vi "New motor Control integrated remodeled with PID.vi"(0 "States":enum16{"RESET ENCODER", "WRITE", "READ", "INIT"}(ring), 1 "Target Speed":T2 {"wTargetSpeed" scale=-1.0..1.0; "yTargetSpeed" scale=-1.0..1.0; "xTargetSpeed" scale=-1.0..1.0}, 3 "Error in":errorcluster) -> (5 "Speed and distance cluster":T1, 6 "Error out":errorcluster)   [LabVIEW 2018]
uses:
  <vilib>/addons/control/pid/pid.llb/PID (DBL).vi
  <vilib>/addons/control/pid/NI_PID_pid.lvlib
panel:
  out "output 3":dbl format="%.2f"
  out "output 2":dbl format="%.2f"
  out "output":dbl format="%.2f"
  out "output variable":dbl
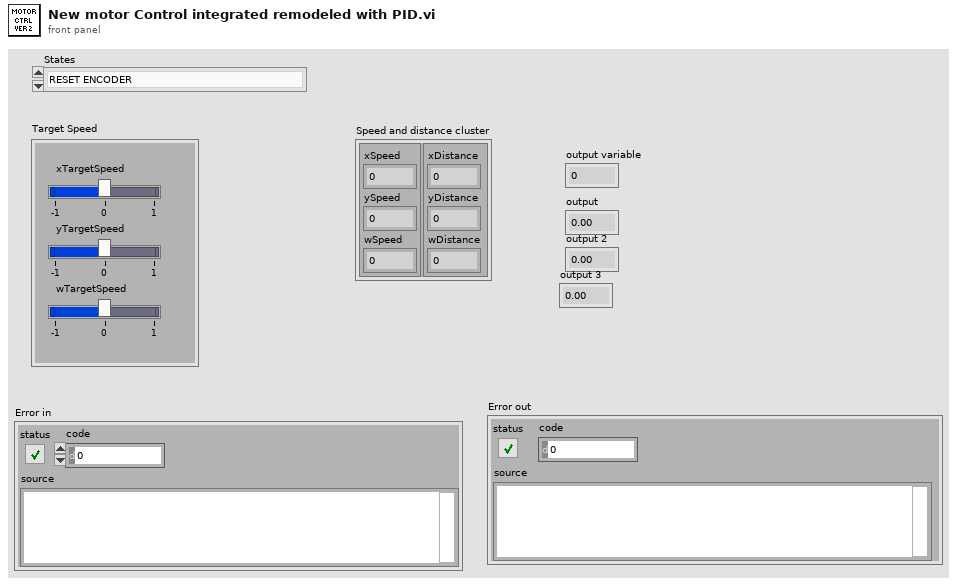
[diagram p1: front panel]
types:
  T1 = cluster{cluster{"xSpeed":dbl, "ySpeed":dbl, "wSpeed":dbl}, cluster{"xDistance":dbl, "yDistance":dbl, "wDistance":dbl}}
  T2 = cluster{"xTargetSpeed":dbl, "yTargetSpeed":dbl, "wTargetSpeed":dbl}
  T3 = cluster{"Encoder 0":dbl, "Encoder 1":dbl, "Encoder 2":dbl}
  T4 = cluster{"proportional gain (Kc)":dbl, "integral time (Ti, min)":dbl, "derivative time (Td, min)":dbl}
  T5 = cluster{"Distance M0 ":dbl, "Distance M1 ":dbl, "Distance M2 ":dbl}
  T6 = cluster{"xDistance":dbl, "yDistance":dbl, "wDistance":dbl}
  T7 = cluster{"xSpeed":dbl, "ySpeed":dbl, "wSpeed":dbl}
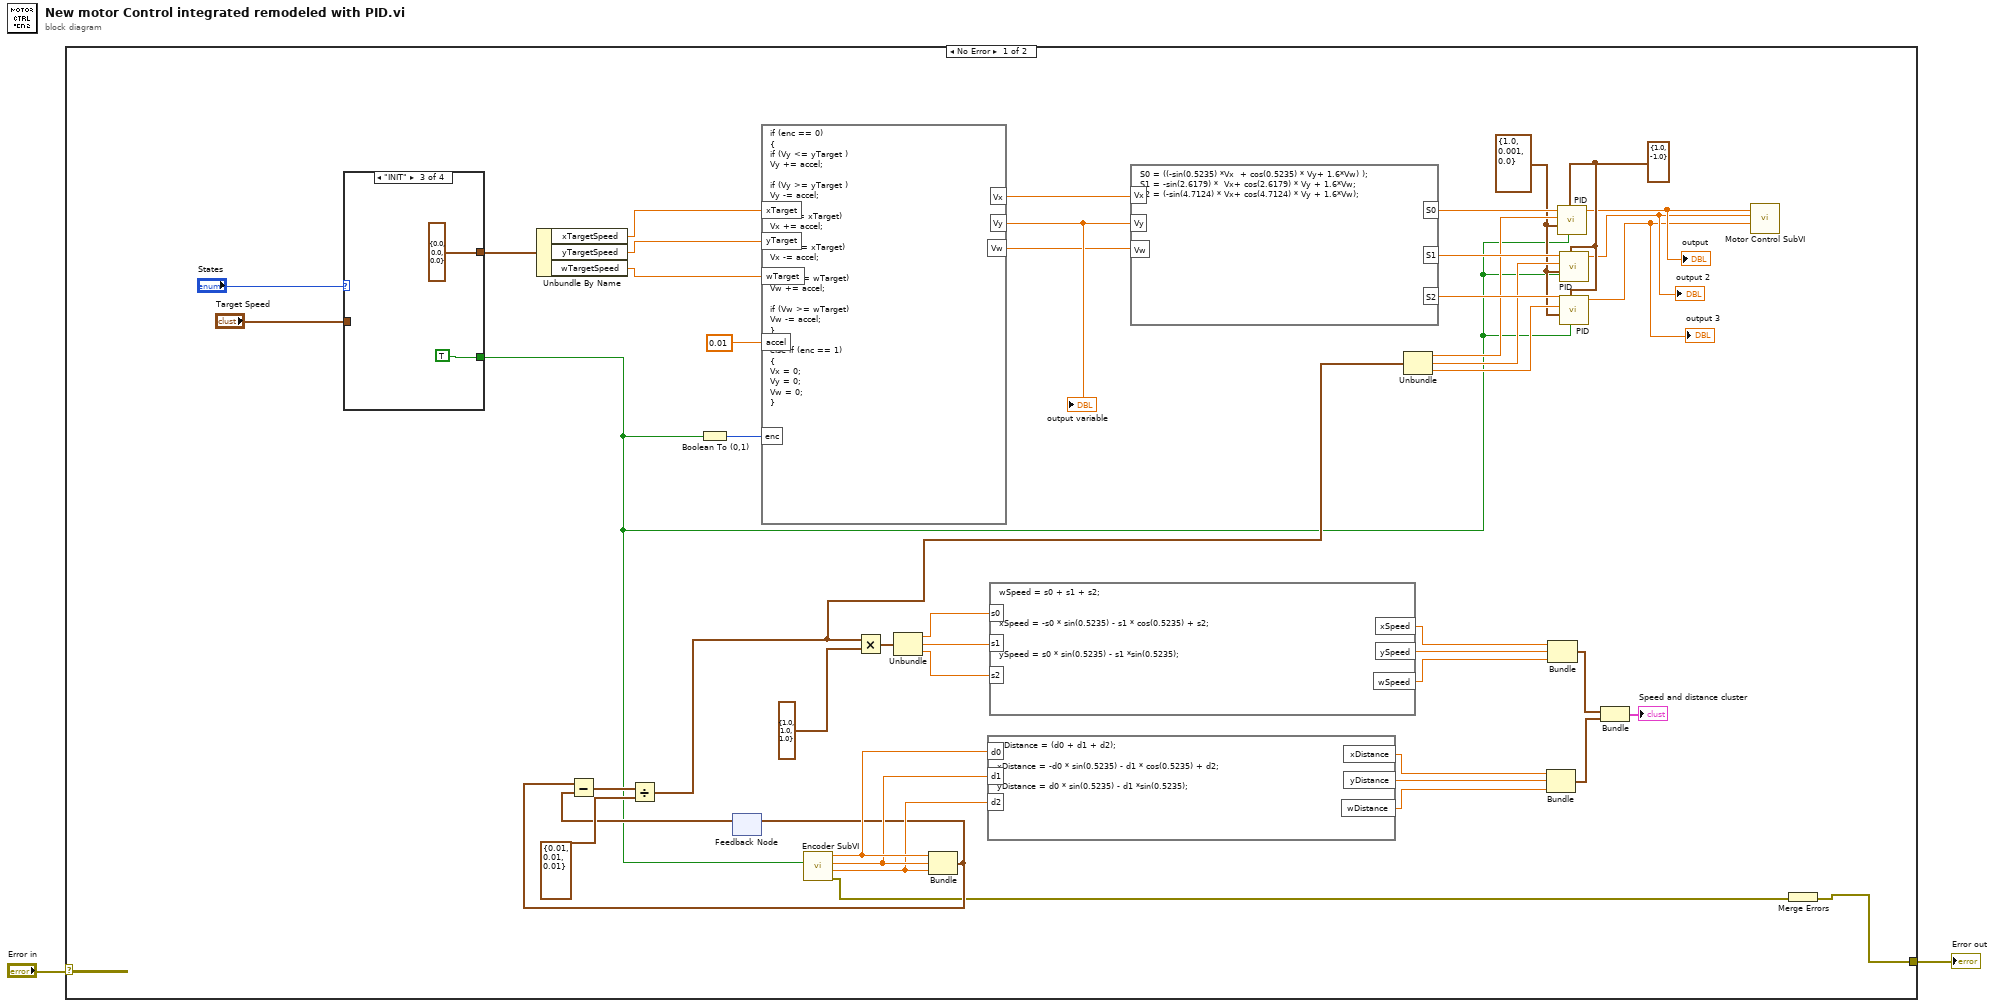
[diagram p0: block diagram]
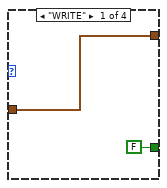
[diagram p2: hidden frame]
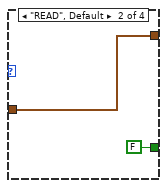
[diagram p3: hidden frame]
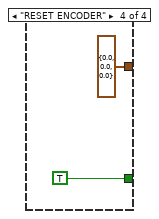
[diagram p4: hidden frame]
diagram:
  n1 = case shown="No Error" "Error in" {
    selector: "Error in" -> [_ w58]
    tunnel: [w49 w58] -> w1
    frame No Error {
      w8 = cluster{"output high":dbl, "output low":dbl} {"output high"=1.0, "output low"=-1.0} ("output range")
      w9 = T4 {"proportional gain (Kc)"=1.0, "integral time (Ti, min)"=0.001, "derivative time (Td, min)"=0.0} ("PID gains")
      n2 = case shown="\"INIT\"" "States" {
        tunnel: "Target Speed" -> [w51 w52 _ _]
        tunnel: [w51 w52 T2 {"xTargetSpeed"=0.0, "yTargetSpeed"=0.0, "wTargetSpeed"=0.0} ("Target Speed") T2 {"xTargetSpeed"=0.0, "yTargetSpeed"=0.0, "wTargetSpeed"=0.0} ("Target Speed")] -> w29
        tunnel: [FALSE ("Reset Encoders") FALSE ("Reset Encoders") TRUE TRUE ("Reset Encoders")] -> w3
        frame "WRITE" {
        }
        frame "READ", Default {
        }
        frame "INIT" {
        }
        frame "RESET ENCODER" {
        }
      }
      n3 = Unbundle By Name(w29) -> ("xTargetSpeed"=w20:dbl, "yTargetSpeed"=w19:dbl, "wTargetSpeed"=w18:dbl)
      n4 = Boolean To (0,1)(Boolean=w3) -> (0, 1=w17:i16)
      n5 = feedback #1() -> (w41:T5)  [unwired: 1 in]
      n6 = formula code="if (enc == 0)\n{\nif (Vy <= yTarget )\nVy += accel;\n\nif (Vy >= yTarget )\nVy -= accel;\n\nif(Vx <= xTarget)\nVx += accel;\n\nif (Vx >= xTarget)\nVx -= accel;\n\nif (Vw <= wTarget)\nVw += accel;\n\nif (Vw >= wTarget)\nVw -= accel;\n}\n\nelse if (enc == 1)\n{\nVx = 0;\nVy = 0;\nVw = 0;\n}"("xTarget"=w20, "yTarget"=w19, "wTarget"=w18, "accel"=0.01 ("input variable"), "enc"=w17) -> ("Vy"=w23:dbl, "Vx"=w24:dbl, "Vw"=w22:dbl)
      "output variable" <- w23
      n7 = call "Encoder SubVI.vi"("Reset Encoders"=w3) -> ("error out"=w26:errorcluster, "Distance M2"=w38:dbl, "Distance M1"=w39:dbl, "Distance M0"=w40:dbl)  [unwired: 7 in]
      n8 = Bundle("Distance M0"=w40, "Distance M1"=w39, "Distance M2"=w38) -> (w32:T5)  [unwired: 1 in]
      n9 = Subtract(x=w32, y=w41) -> (x-y=w48:T5)
      n10 = Divide(x=w48, y=T3 {"Encoder 0"=0.01, "Encoder 1"=0.01, "Encoder 2"=0.01}) -> (x/y=w7:cluster{dbl, dbl, dbl})
      n11 = feedback-in #1(w32) -> ()
      n12 = Multiply(x=w7, y=cluster{dbl, dbl, dbl} {1.0, 1.0, 1.0}) -> (x*y=w13:cluster{dbl, dbl, dbl})
      n13 = Unbundle(w13) -> (w33:dbl, w43:dbl, w42:dbl)
      n14 = formula code="wDistance = (d0 + d1 + d2);\n\nxDistance = -d0 * sin(0.5235) - d1 * cos(0.5235) + d2;\n\nyDistance = d0 * sin(0.5235) - d1 *sin(0.5235);"("d0"=w40, "d1"=w39, "d2"=w38) -> ("xDistance"=w37:dbl, "wDistance"=w35:dbl, "yDistance"=w36:dbl)
      n15 = formula code="wSpeed = s0 + s1 + s2;\n\n\nxSpeed = -s0 * sin(0.5235) - s1 * cos(0.5235) + s2;\n\n\nySpeed = s0 * sin(0.5235) - s1 *sin(0.5235);"("s0"=w33, "s1"=w43, "s2"=w42) -> ("xSpeed"=w45:dbl, "ySpeed"=w46:dbl, "wSpeed"=w44:dbl)
      n16 = formula code="S0 = ((-sin(0.5235) *Vx  + cos(0.5235) * Vy+ 1.6*Vw) );\nS1 = -sin(2.6179) *  Vx+ cos(2.6179) * Vy + 1.6*Vw;\nS2 = (-sin(4.7124) * Vx+ cos(4.7124) * Vy + 1.6*Vw);"("Vx"=w24, "Vy"=w23, "Vw"=w22) -> ("S0"=w16:dbl, "S1"=w15:dbl, "S2"=w14:dbl)
      n17 = Unbundle(w7) -> (w12:dbl, w11:dbl, w10:dbl)
      n18 = Bundle("xDistance"=w37, "yDistance"=w36, "wDistance"=w35) -> (w28:T6)  [unwired: 1 in]
      n19 = Bundle("xSpeed"=w45, "ySpeed"=w46, "wSpeed"=w44) -> (w25:T7)  [unwired: 1 in]
      n20 = call-poly <vilib>:"PID.vi"("reinitialize? (F)"=w3, "output range"=w8, "PID gains"=w9, "process variable"=w12, "setpoint"=w16) -> ("output"=w6:dbl)  [unwired: 5 in, 1 out]
      "output" <- w6
      n21 = call-poly <vilib>:"PID.vi"("reinitialize? (F)"=w3, "output range"=w8, "PID gains"=w9, "process variable"=w11, "setpoint"=w15) -> ("output"=w5:dbl)  [unwired: 5 in, 1 out]
      "output 2" <- w5
      n22 = call-poly <vilib>:"PID.vi"("reinitialize? (F)"=w3, "output range"=w8, "PID gains"=w9, "process variable"=w10, "setpoint"=w14) -> ("output"=w4:dbl)  [unwired: 5 in, 1 out]
      "output 3" <- w4
      n23 = Bundle(w25, w28) -> (→"Speed and distance cluster":T1)  [unwired: 1 in]
      n24 = call "Motor Control SubVI.vi"("Speed M2"=w4, "Speed M1"=w5, "Speed M0"=w6) -> ()  [unwired: 8 in, 1 out]
      n25 = Merge Errors(w26) -> (w49:errorcluster)
    }
    frame Error {
    }
  }
  "Error out" <- w1
